vi "Write PAS Data.vi"(8 "error in (no error)":errorcluster, 10 "DataIn":refnum<class "Data.lvclass">, 11 "Data MSG in":refnum<class "Data MSG.lvclass">) -> (0 "error out":errorcluster, 3 "Data MSG out":refnum<class "Data MSG.lvclass">)   [LabVIEW 2014, in "Instrument Library.lvlib" / "Data MSG.lvclass"]
uses:
  Data MSG.lvclass
  reusable/Data/Data.lvclass
  Data MSG.lvclass/Data MSG.ctl
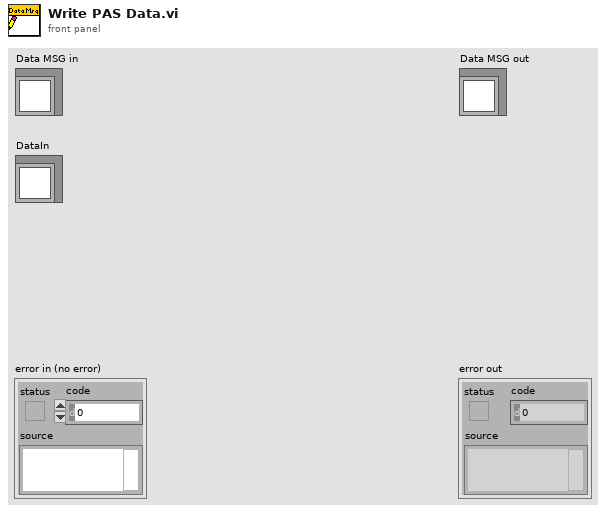
[diagram p1: front panel]
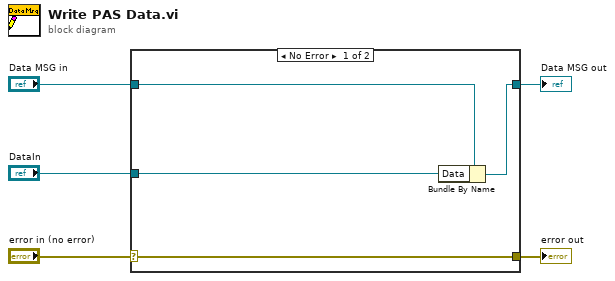
[diagram p0: block diagram]
diagram:
  n1 = case shown="No Error" "error in (no error)" {
    selector: "error in (no error)" -> [w9 w10]
    tunnel: [w9 w10] -> w4
    tunnel: [w7 w11] -> w2
    tunnel: "Data MSG in" -> [w8 w11]
    tunnel: "DataIn" -> [w6 _]
    frame No Error {
      n2 = Bundle By Name(cluster=w8, "Data"=w6) -> (w7:refnum<class "Data MSG.lvclass">)
    }
    frame Error {
    }
  }
  "error out" <- w4
  "Data MSG out" <- w2
